vi "mkSetExposureGainOffset.vi"(7 "Set? (F)":bool, 8 "Gain [1-4]":sgl, 9 "Offset":i16, 10 "Exposure time":i32, 11 "IMAQ Refnum in":refnum<k11>) -> (0 "Gain":dbl, 1 "Offset":u32, 2 "Exposure time":i32, 3 "IMAQ Refnum out":refnum<k11>, 4 "Max exposure time":i32, 6 "Min exposure time":i32)   [LabVIEW 2011]
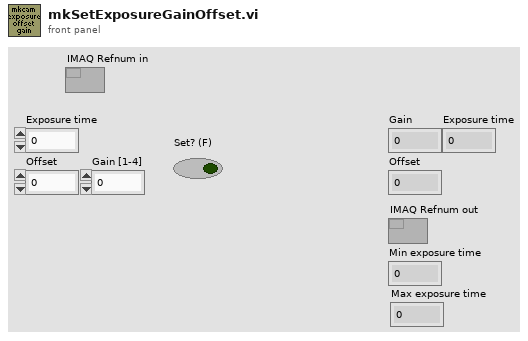
[diagram p1: front panel]
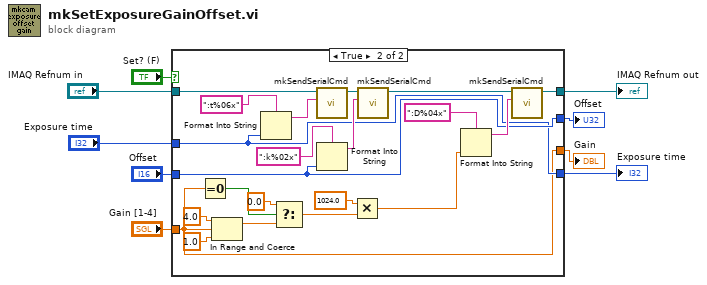
[diagram p0: block diagram]
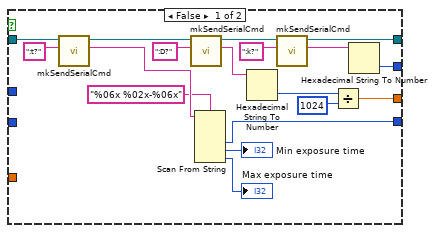
[diagram p2: hidden frame]
diagram:
  n1 = case shown="True" "Set? (F)" {
    tunnel: "IMAQ Refnum in" -> [w27 w48]
    tunnel: [w24 w37] -> w7
    tunnel: "Exposure time" -> [_ w29]
    tunnel: "Offset" -> [_ w30]
    tunnel: "Gain [1-4]" -> [_ w28]
    tunnel: [w12 w28] -> w3
    tunnel: [w11 w29] -> w2
    tunnel: [w10 w30] -> w1
    frame False {
      n2 = call "mkSendSerialCmd.vi"("String"=":t?", "IMAQ Refnum in"=w27) -> ("String Read"=w18:string, "IMAQ Refnum out"=w26:refnum<k11>)  [unwired: 6 in, 2 out]
      n3 = call "mkSendSerialCmd.vi"("String"=":D?", "IMAQ Refnum in"=w26) -> ("String Read"=w19:string, "IMAQ Refnum out"=w25:refnum<k11>)  [unwired: 6 in, 2 out]
      n4 = Scan From String(format string="%06x %02x-%06x", input string=w18) -> (output 1=w11:i32, output 2=→"Min exposure time":i32, output 3=→"Max exposure time":i32)  [unwired: 5 in, 3 out]
      n5 = Hexadecimal String To Number(string=w19) -> (number=w14:u32)  [unwired: 2 in, 1 out]
      n6 = call "mkSendSerialCmd.vi"("String"=":k?", "IMAQ Refnum in"=w25) -> ("String Read"=w20:string, "IMAQ Refnum out"=w24:refnum<k11>)  [unwired: 6 in, 2 out]
      n7 = Divide(x=w14, y=u32 1024) -> (x/y=w12:dbl)
      n8 = Hexadecimal String To Number(string=w20) -> (number=w10:u32)  [unwired: 2 in, 1 out]
    }
    frame True {
      n9 = Equal To 0?(x=w28) -> (x = 0?=w34:bool)
      n10 = In Range and Coerce(upper limit=4.0, x=w28, lower limit=1.0 ("x")) -> (coerced(x)=w32:dbl)  [unwired: 1 out]
      n11 = Format Into String(format string=":t%06x", w29) -> (resulting string=w46:string)  [unwired: 2 in, 1 out]
      n12 = Select(t=0.0, s=w34, f=w32) -> (s? t:f=w31:dbl)
      n13 = call "mkSendSerialCmd.vi"("String"=w46, "IMAQ Refnum in"=w48) -> ("IMAQ Refnum out"=w38:refnum<k11>)  [unwired: 6 in, 3 out]
      n14 = Format Into String(format string=":k%02x", w30) -> (resulting string=w39:string)  [unwired: 2 in, 1 out]
      n15 = Multiply(x=1024.0, y=w31) -> (x*y=w42:dbl)
      n16 = call "mkSendSerialCmd.vi"("String"=w39, "IMAQ Refnum in"=w38) -> ("IMAQ Refnum out"=w40:refnum<k11>)  [unwired: 6 in, 3 out]
      n17 = Format Into String(format string=":D%04x", w42) -> (resulting string=w41:string)  [unwired: 2 in, 1 out]
      n18 = call "mkSendSerialCmd.vi"("String"=w41, "IMAQ Refnum in"=w40) -> ("IMAQ Refnum out"=w37:refnum<k11>)  [unwired: 6 in, 3 out]
    }
  }
  "IMAQ Refnum out" <- w7
  "Gain" <- w3
  "Offset" <- w1
  "Exposure time" <- w2
